vi "Write Age Wrapper.vi"(8 "error in (no error)":errorcluster, 10 "age":dbl, 11 "myClass in":refnum<class "myClass.lvclass">) -> (0 "error out":errorcluster, 3 "myClass out":refnum<class "myClass.lvclass">)   [LabVIEW 2011]
uses:
  myClass.lvclass
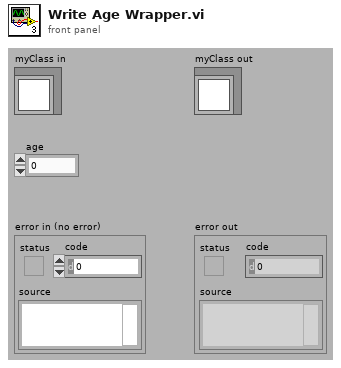
[diagram p1: front panel]
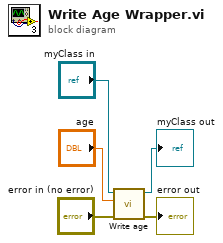
[diagram p0: block diagram]
diagram:
  n1 = call-dynamic "Write age.vi"("error in (no error)"="error in (no error)", "age"="age", "myClass in"="myClass in") -> ("error out"=→"error out":errorcluster, "myClass out"=→"myClass out":refnum<class "myClass.lvclass">)  [unwired: 7 in]
